vi "v6.0.vi"() -> ()   [LabVIEW 2018]
uses:
  <vilib>/DAQmx/read.llb/DAQmx Read (Analog 1D DBL NChan 1Samp).vi
  <extravilib>/ChannelInstances/Lossy Stream-c(a[.](c(dbl,dbl,dbl,dbl)),stamp,a[.](dbl),c(dbl,dbl,dbl,dbl,dbl,dbl,dbl))/Read With Abort.vi
  <extravilib>/ChannelInstances/High Speed Stream-c(a[.](c(dbl,dbl,dbl,dbl)),stamp,a[.](dbl),c(dbl,dbl,dbl,dbl,dbl,dbl,dbl))/_Read For Replicate.vi
  <extravilib>/ChannelInstances/Lossy Stream-c(a[.](c(dbl,dbl,dbl,dbl)),stamp,a[.](dbl),c(dbl,dbl,dbl,dbl,dbl,dbl,dbl))/Write With Abort.vi
  <extravilib>/ChannelInstances/Lossy Stream-c(a[.](c(dbl,dbl,dbl,dbl)),stamp,a[.](dbl),c(dbl,dbl,dbl,dbl,dbl,dbl,dbl))/EndpointRead.vi
  <extravilib>/ChannelInstances/Lossy Stream-c(a[.](c(dbl,dbl,dbl,dbl)),stamp,a[.](dbl),c(dbl,dbl,dbl,dbl,dbl,dbl,dbl))/Endpoint.vi
  <extravilib>/ChannelInstances/Lossy Stream-c(a[.](c(dbl,dbl,dbl,dbl)),stamp,a[.](dbl),c(dbl,dbl,dbl,dbl,dbl,dbl,dbl))/Instantiate.vi
  <extravilib>/ChannelInstances/Lossy Stream-c(a[.](c(dbl,dbl,dbl,dbl)),stamp,a[.](dbl),c(dbl,dbl,dbl,dbl,dbl,dbl,dbl))/)Channel.vi
  <resource>/ChannelSupport/_ChannelSupport/WaitIfNeeded.vi
  <extravilib>/ChannelInstances/High Speed Stream-c(a[.](c(dbl,dbl,dbl,dbl)),stamp,a[.](dbl),c(dbl,dbl,dbl,dbl,dbl,dbl,dbl))/Instantiate.vi
  <extravilib>/ChannelInstances/High Speed Stream-c(a[.](c(dbl,dbl,dbl,dbl)),stamp,a[.](dbl),c(dbl,dbl,dbl,dbl,dbl,dbl,dbl))/)Channel.vi
  <extravilib>/ChannelInstances/High Speed Stream-c(a[.](c(dbl,dbl,dbl,dbl)),stamp,a[.](dbl),c(dbl,dbl,dbl,dbl,dbl,dbl,dbl))/Abort Signal/Init Signal.vi
  <vilib>/Utility/file.llb/Write Delimited Spreadsheet (string).vi
  <vilib>/DAQmx/create/channels.llb/DAQmx Create Channel (AI-Temperature-Thermocouple).vi
  <vilib>/DAQmx/configure/timing.llb/DAQmx Timing (Sample Clock).vi
  <vilib>/DAQmx/miscellaneous.llb/DAQmx Fill In Error Info.vi
  <extravilib>/ChannelInstances/High Speed Stream-c(a[.](c(dbl,dbl,dbl,dbl)),stamp,a[.](dbl),c(dbl,dbl,dbl,dbl,dbl,dbl,dbl)).lvlib
  <resource>/objmgr/daqmx.rc
  <extravilib>/ChannelInstances/Lossy Stream-c(a[.](c(dbl,dbl,dbl,dbl)),stamp,a[.](dbl),c(dbl,dbl,dbl,dbl,dbl,dbl,dbl)).lvlib
panel:
  in  "Line Controls\n(Don't Delete)":enum32{"Flowrate", "Temperatures", "Pressures"}(tab)
  in  "Line Flowrate Control":T1 {"Line 5" scale=0.0..10.0; "Line 4" scale=0.0..10.0; "Line 3" scale=0.0..10.0; "Line 2" scale=0.0..10.0; "Line 1" scale=0.0..10.0}
  in  "Temperatures Control":T1 {"Line 5" scale=0.0..10.0; "Line 4" scale=0.0..10.0; "Line 3" scale=0.0..10.0; "Line 2" scale=0.0..10.0; "Line 1" scale=0.0..10.0}
  in  "Pressure Controls":T1 {"Line 5" scale=0.0..10.0; "Line 4" scale=0.0..10.0; "Line 3" scale=0.0..10.0; "Line 2" scale=0.0..10.0; "Line 1" scale=0.0..10.0}
  out "Thermal Power [kJ/s]":dbl
  out "Equivalence Ratio":dbl
  out "Total Air Flow Required for \nStoichiometric Combustion":dbl
  out "Mixture AFR":dbl
  out "Total Fuel Flow [g/s]":dbl
  out "Total Air Flow [g/s]":dbl
  in  "Rig Temperature Tab Box\n(Don't Delete)":enum32{"Rig Temps Live", "Alarm Thresholds"}(tab)
  out "Rig Temperatures":T2
  in  "Rig Alarm Thresholds":T2
  out "DAQ Current Time":timestamp format="%<%X>T"
  in  "UI Refresh Rate (Hz)":u32=1 min=1 max=500 step=1
  out "Line Pressures":T3(graph)
  out "Line Temperatures":T3(graph)
  in  "Species List":string[][](table)=[["Custom", "9999999999", ""], ["Methanol", "6.47", "19.93"], ["Butanol", "11.2", "33.075"], ["Propane", "15.67", "46.35"], ["Methane", "13.19", "50.00"], ["Hydrogen", "34.3", "119.96"], ["Ammonia", "6.0466", "22.5"], ["Pentane", "15.32", "45.36"], ["Butane", "14.98", "45.75"], ["Hexane", "15.24", "44.75"], ["Ethanol", "9", "26.70"], ["Empty (Not Used)", "0", "0"]]
  in  "Lines Tab Control\n(Don't delete)":enum32{"Live Data", "AFR Info", "Setup Lines"}(tab)
  out "Flowrate Data":T4(array[cluster])
  out "AFR Display":T5(array[cluster])
  in  "Line Setup":T6(array[cluster])
  out "Actual Sample Rate":dbl
  out "Export Timestamp":timestamp format="%<%H:%M:%S>T"
  out "UI Timestamp":timestamp format="%<%X\n%x>T"
  in  "file path (dialog if empty)":path
  out "Export Loop Status":T7(ring)
  in  "Start Recording?":bool
  in  "Stop Recording?":bool
  out "Aquisition\nLoop Status":T8(ring)
  in  "OK Button":bool
  in  "DAQ Properties":cluster{"Sample Rate [Hz]":dbl}={"Sample Rate [Hz]"=1.0} {"Sample Rate [Hz]" min=1.0 max=500.0 step=1.0}
  # "Rig Temperatures [ °C]"
  # "Rig Alarm Thresholds [ °C]"
  # "Live \n Live Line Data"
  # "Air-to-Fuel Ratios for each Line"
  # "Line Setup"
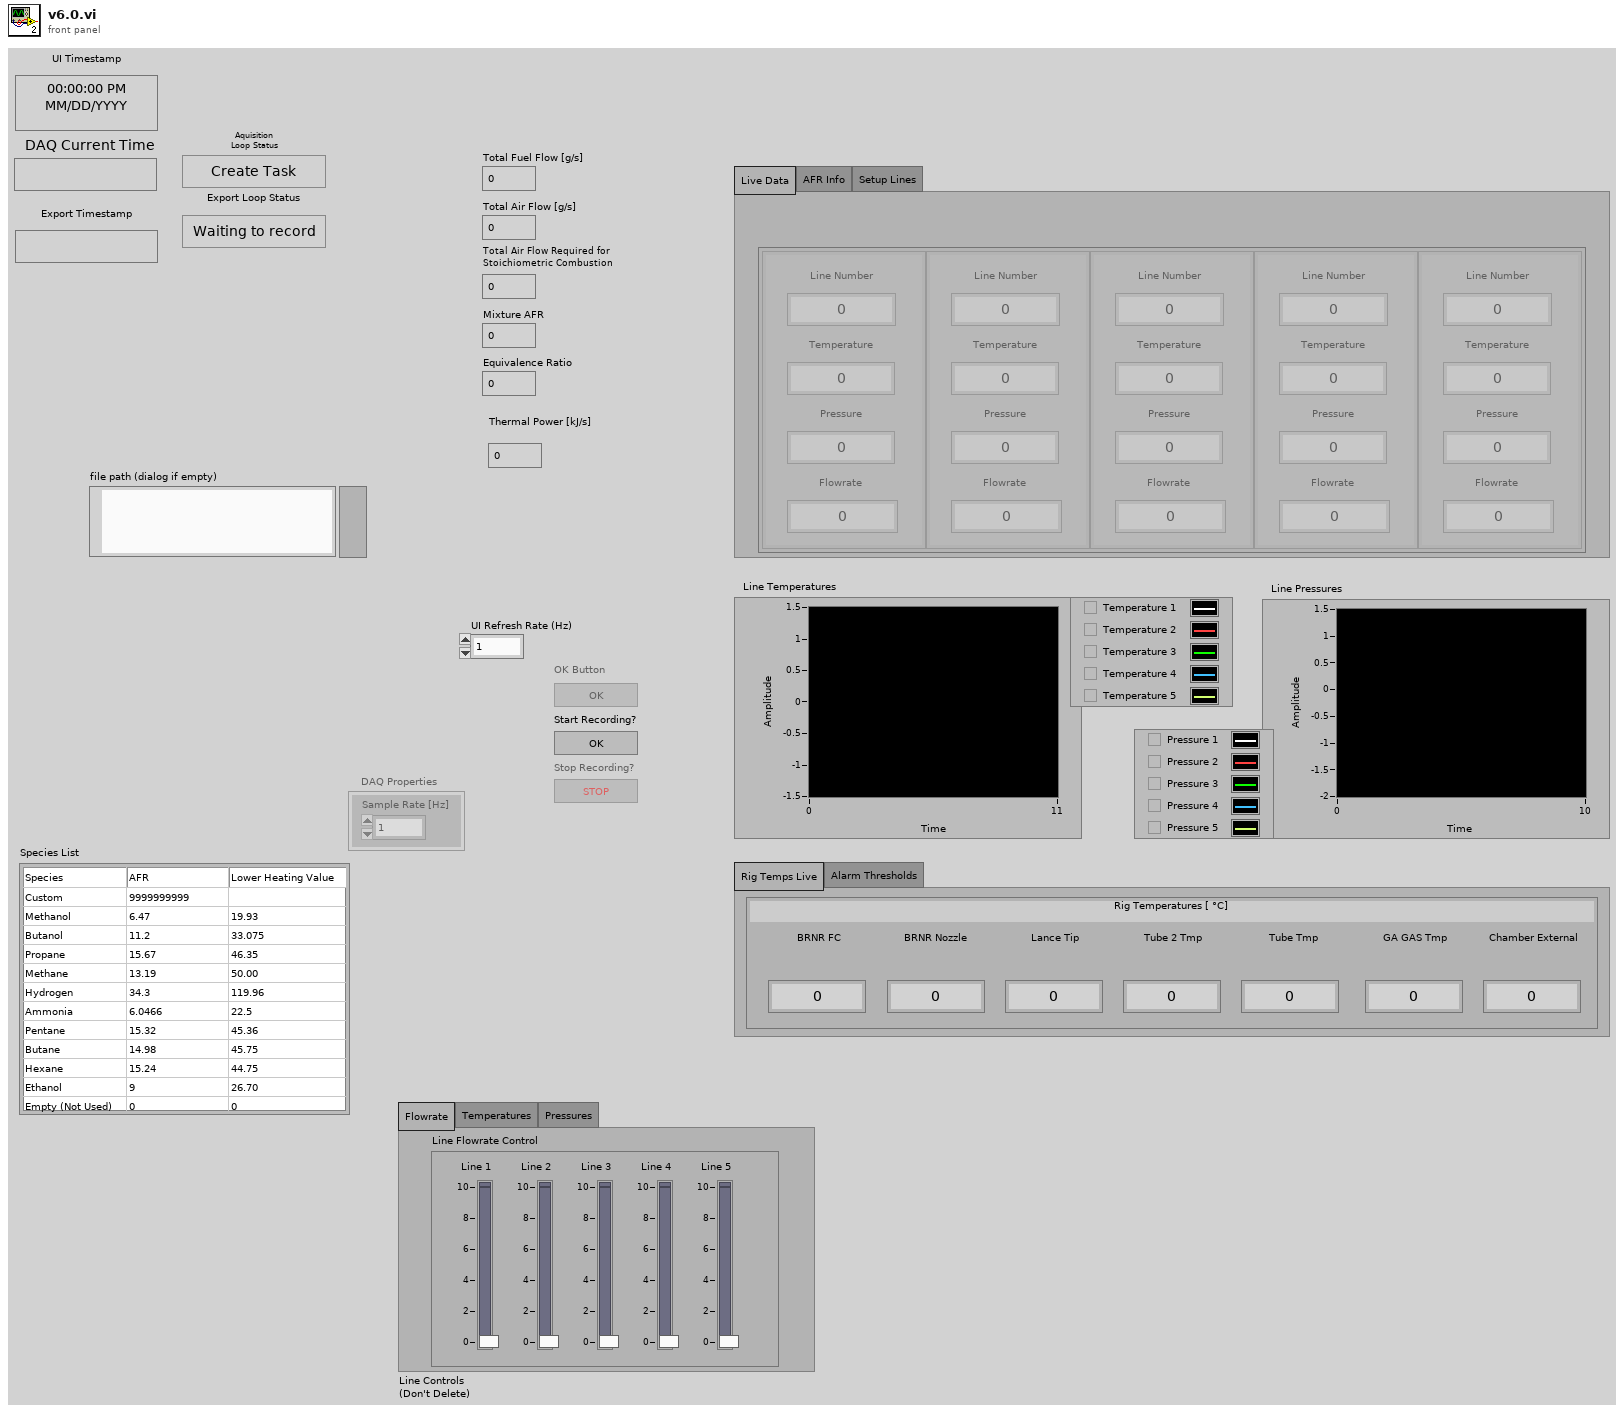
[diagram p1: front panel]
types:
  T1 = cluster{"Line 1":dbl, "Line 2":dbl, "Line 3":dbl, "Line 4":dbl, "Line 5":dbl}
  T2 = cluster{"BRNR FC":dbl, "BRNR Nozzle":dbl, "Lance Tip":dbl, "Tube 2 Tmp":dbl, "Tube Tmp":dbl, "GA GAS Tmp":dbl, "Chamber External":dbl}
  T3 = cluster{"[0]":dbl, "[1]":dbl, "[2]":dbl, "[3]":dbl, "[4]":dbl}
  T4 = cluster{"Line Number":dbl, "Temperature":dbl, "Pressure":dbl, "Flowrate":dbl}[]
  T5 = cluster{"Line Number":i32, "AFR":dbl, "Species":enum16{"Empty (Not used)", "Custom", "Air", "Methanol", "Ethanol", "Butanol", "Propane", "Methane", "Hydrogen", "Pentane", "Butane", "Hexane"}}[]
  T6 = cluster{"Custom AFR":dbl, "Species":enum16{"Empty (Not used)", "Custom", "Air", "Methanol", "Ethanol", "Butanol", "Propane", "Methane", "Hydrogen", "Pentane", "Butane", "Hexane"}, "Custom Lower Heating Value [kJ/kg]":dbl}[]
  T7 = enum16{"Waiting to record", "Creating Spreadsheet", "Recording", "Finished Recording"}
  T8 = enum16{"Create Task", "Change Settings", "Check Settings", "Read Data", "End Task"}
  T9 = enum8{"Enabled", "Disabled", "Disabled and Grayed Out"}
  T10 = cluster{"Flowrate Data":cluster{"Line Number":dbl, "Temperature":dbl, "Pressure":dbl, "Flowrate":dbl}[], "Current Time":timestamp, "DAQmx Data":dbl[], "Rig Temperatures":cluster{"BRNR FC":dbl, "BRNR Nozzle":dbl, "Lance Tip":dbl, "Tube 2 Tmp":dbl, "Tube Tmp":dbl, "GA GAS Tmp":dbl, "Chamber External Temp":dbl}}
  T11 = cluster{"BRNR FC":dbl, "BRNR Nozzle":dbl, "Lance Tip":dbl, "Tube 2 Tmp":dbl, "Tube Tmp":dbl, "GA GAS Tmp":dbl, "Chamber External Temp":dbl}
  T12 = typedef "High Speed Stream-c(a[.](c(dbl,dbl,dbl,dbl)),stamp,a[.](dbl),c(dbl,dbl,dbl,dbl,dbl,dbl,dbl)).lvlib/)Channel.ctl" = refnum<queue>
  T13 = typedef "Lossy Stream-c(a[.](c(dbl,dbl,dbl,dbl)),stamp,a[.](dbl),c(dbl,dbl,dbl,dbl,dbl,dbl,dbl)).lvlib/)Channel.ctl" = refnum<queue>
  T14 = cluster{"Line":i32, "AFR":dbl, "Species":enum16{"Empty (Not used)", "Custom", "Air", "Methanol", "Ethanol", "Butanol", "Propane", "Methane", "Hydrogen", "Pentane", "Butane", "Hexane"}}
  T15 = enum16{"Empty (Not used)", "Custom", "Air", "Methanol", "Ethanol", "Butanol", "Propane", "Methane", "Hydrogen", "Pentane", "Butane", "Hexane"}
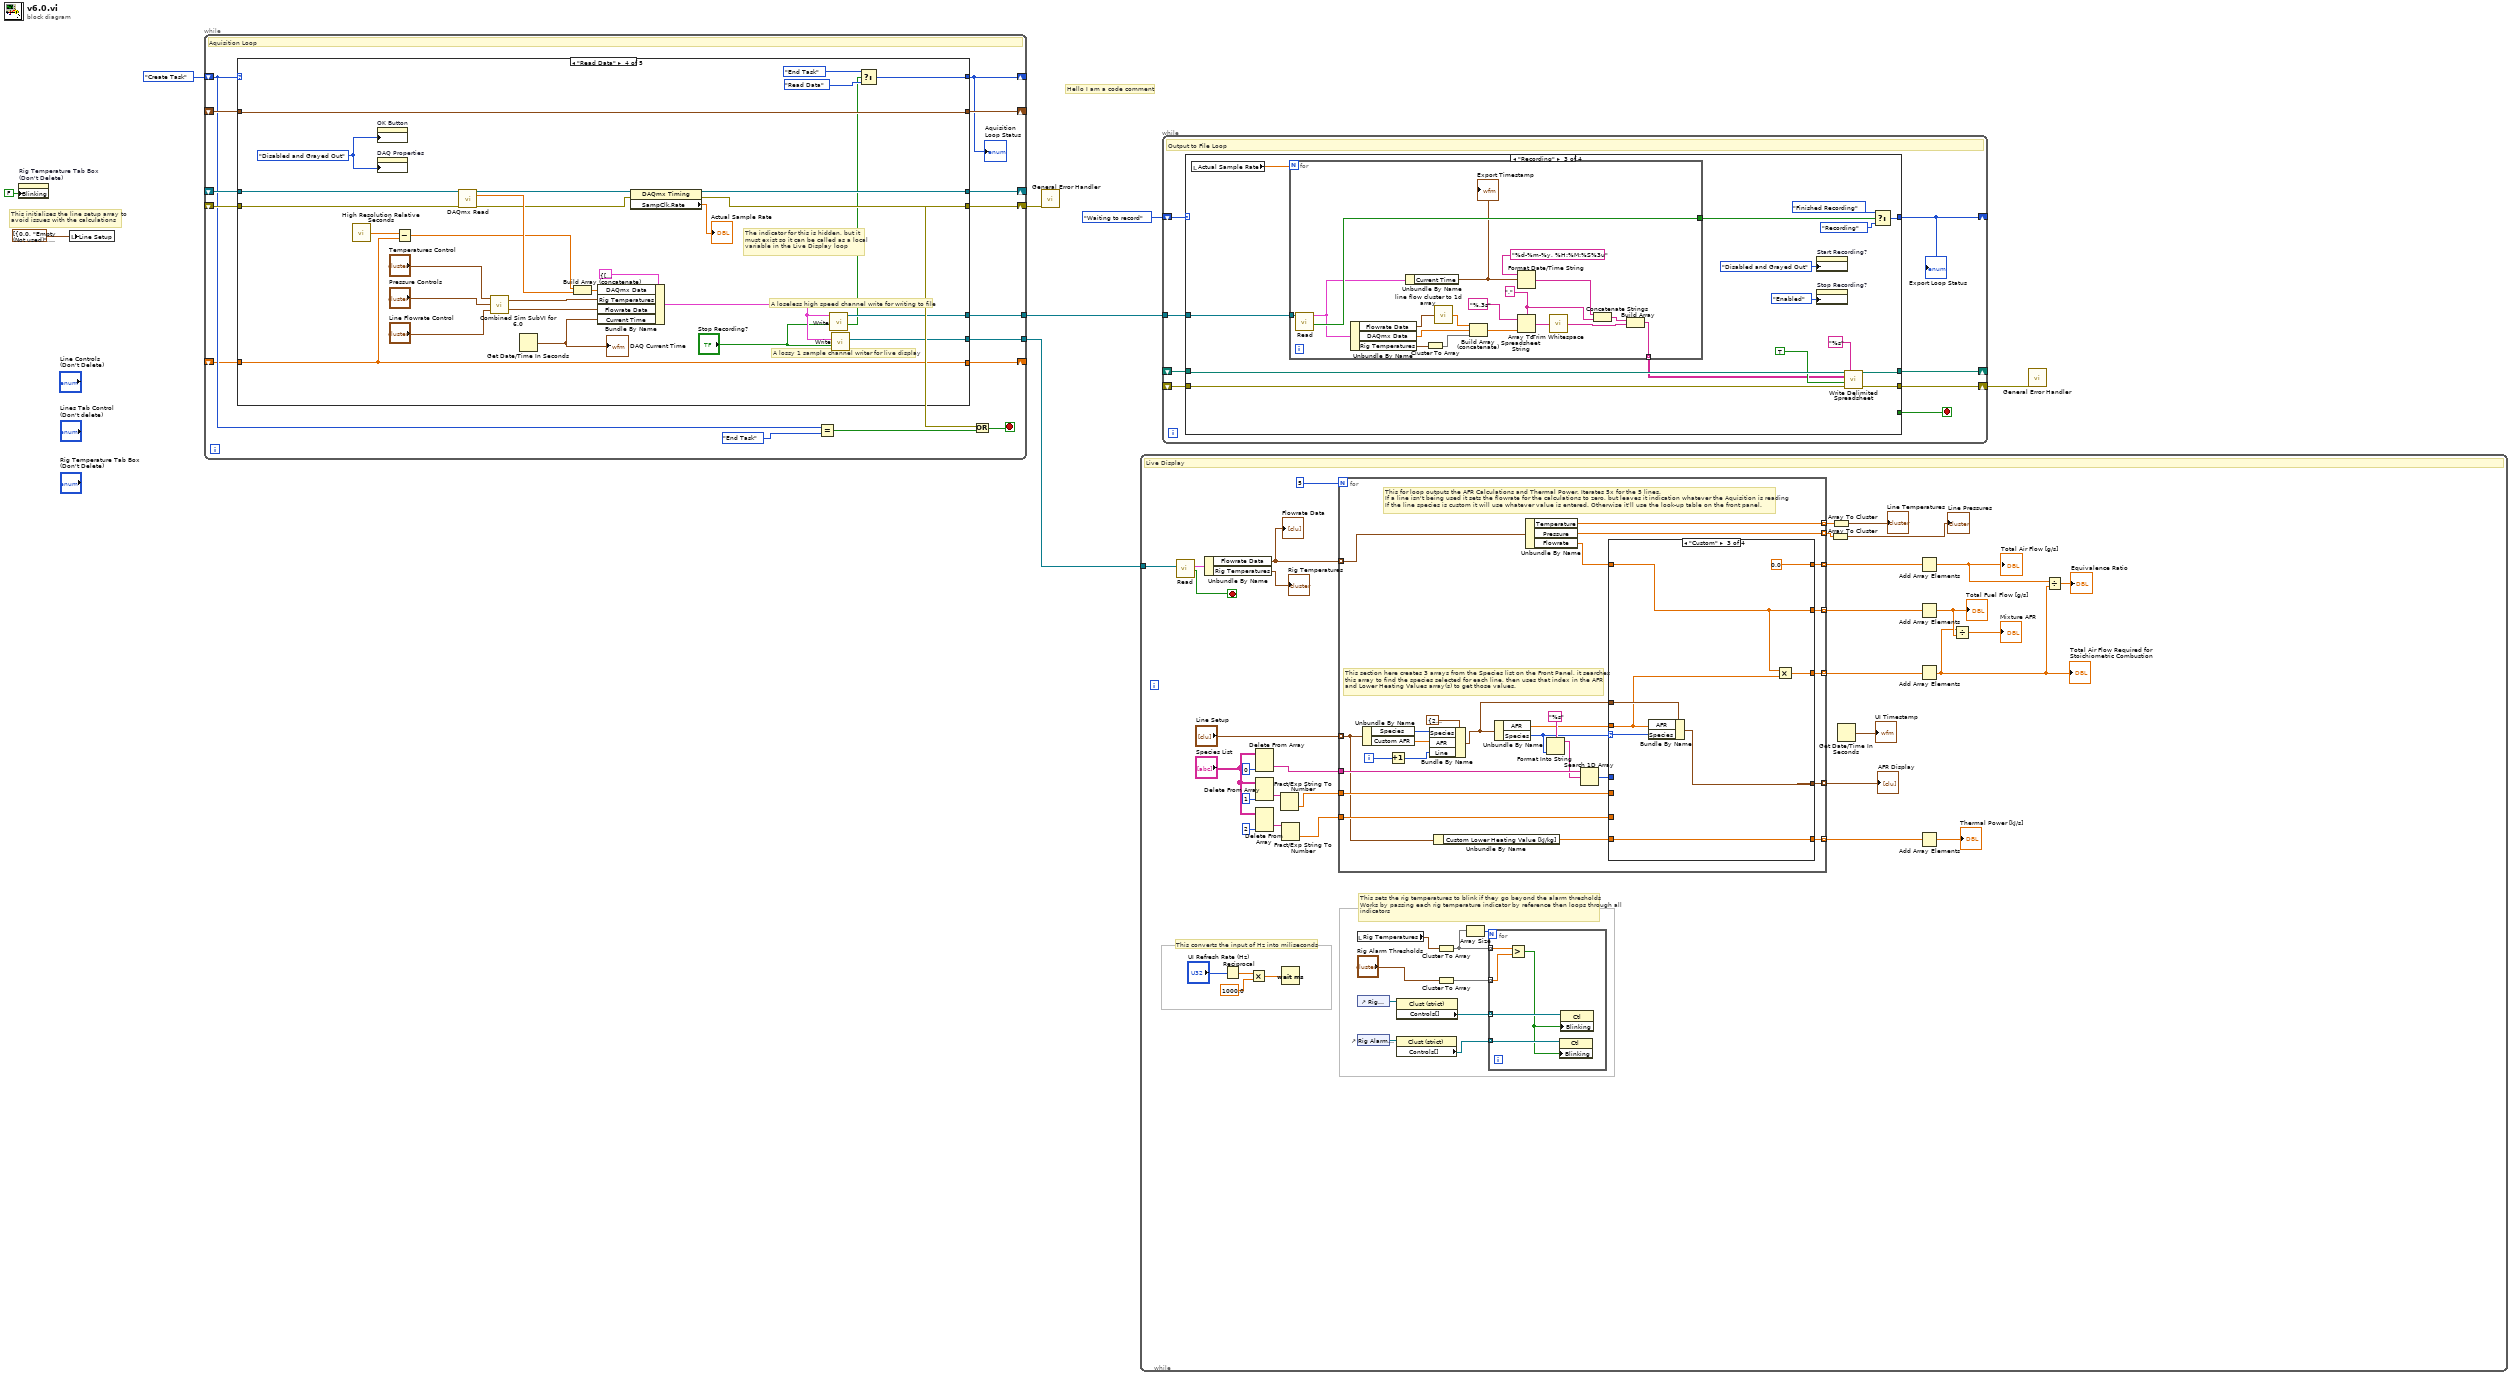
[diagram p0: block diagram]
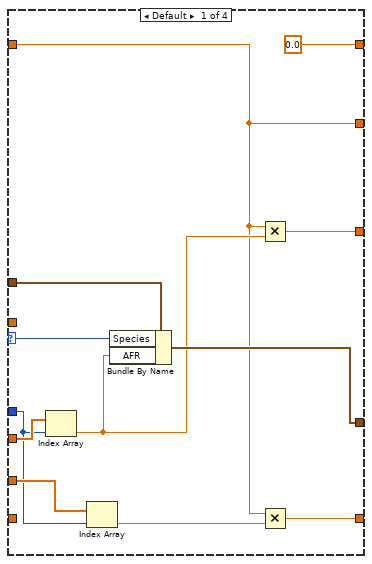
[diagram p2: hidden frame]
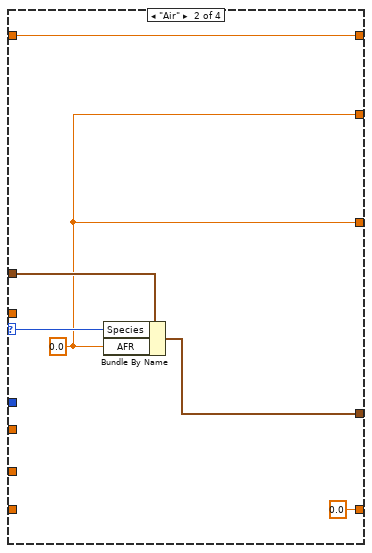
[diagram p3: hidden frame]
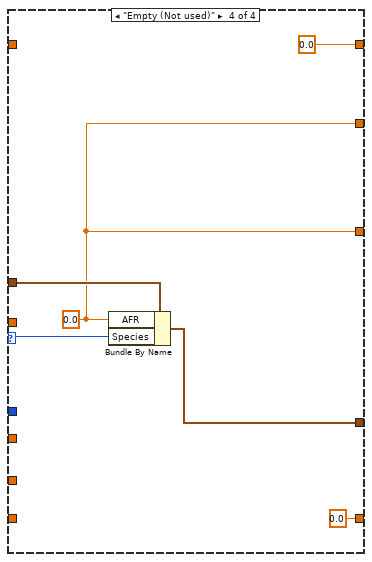
[diagram p4: hidden frame]
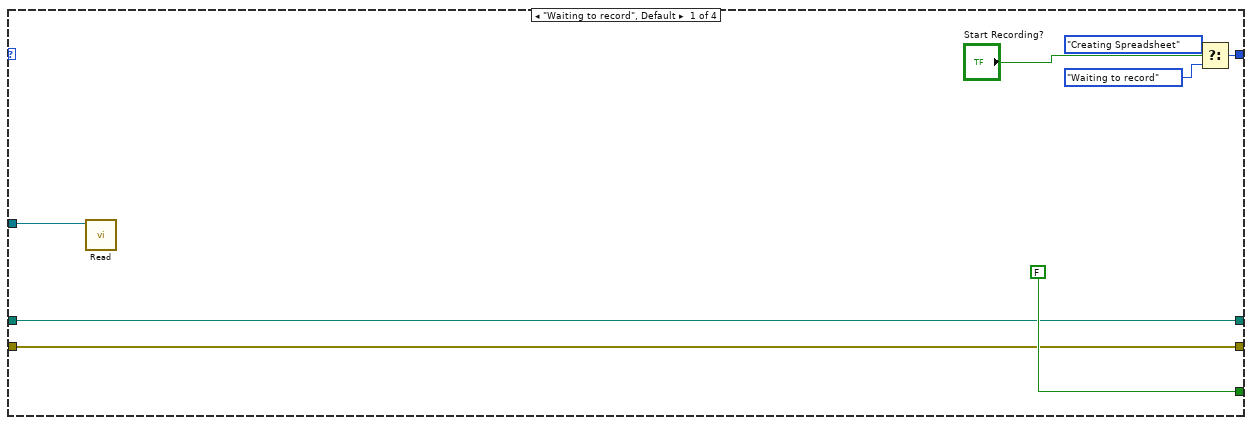
[diagram p5: hidden frame]
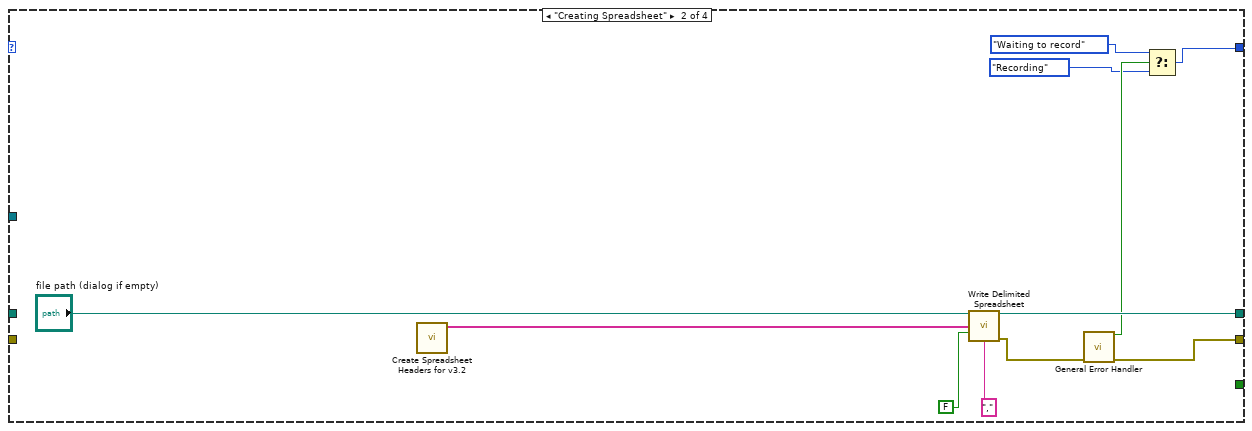
[diagram p6: hidden frame]
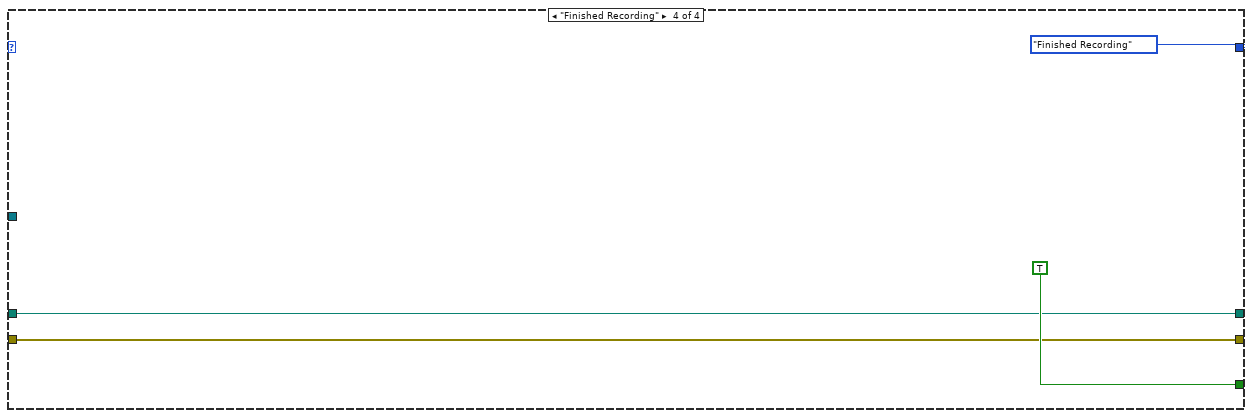
[diagram p7: hidden frame]
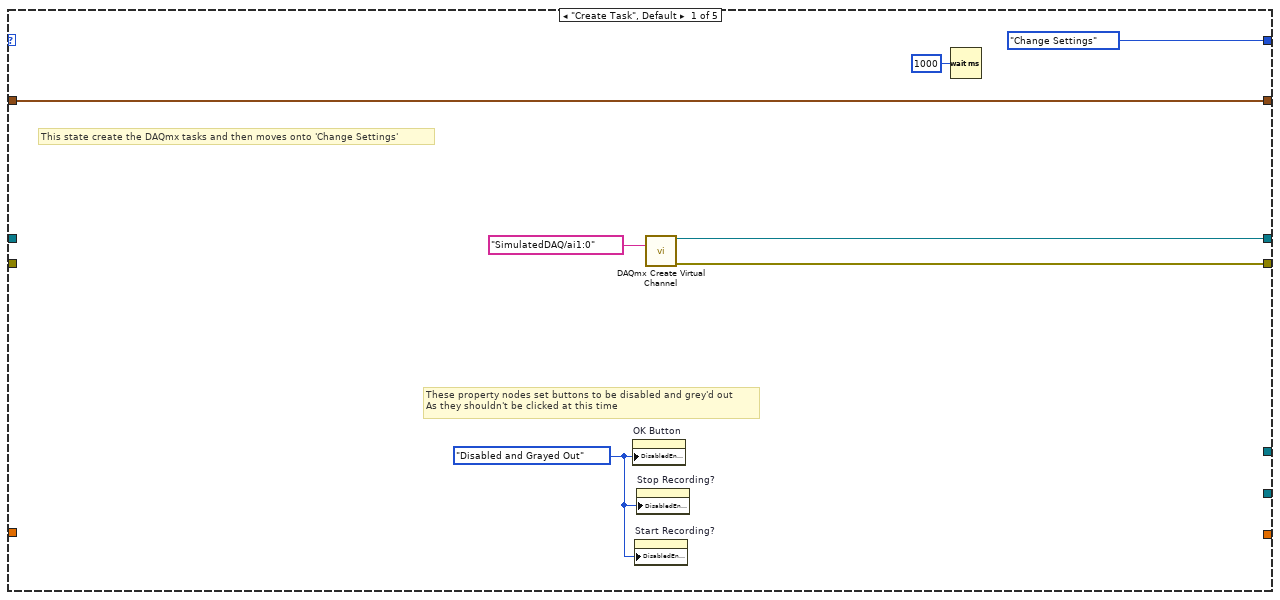
[diagram p8: hidden frame]
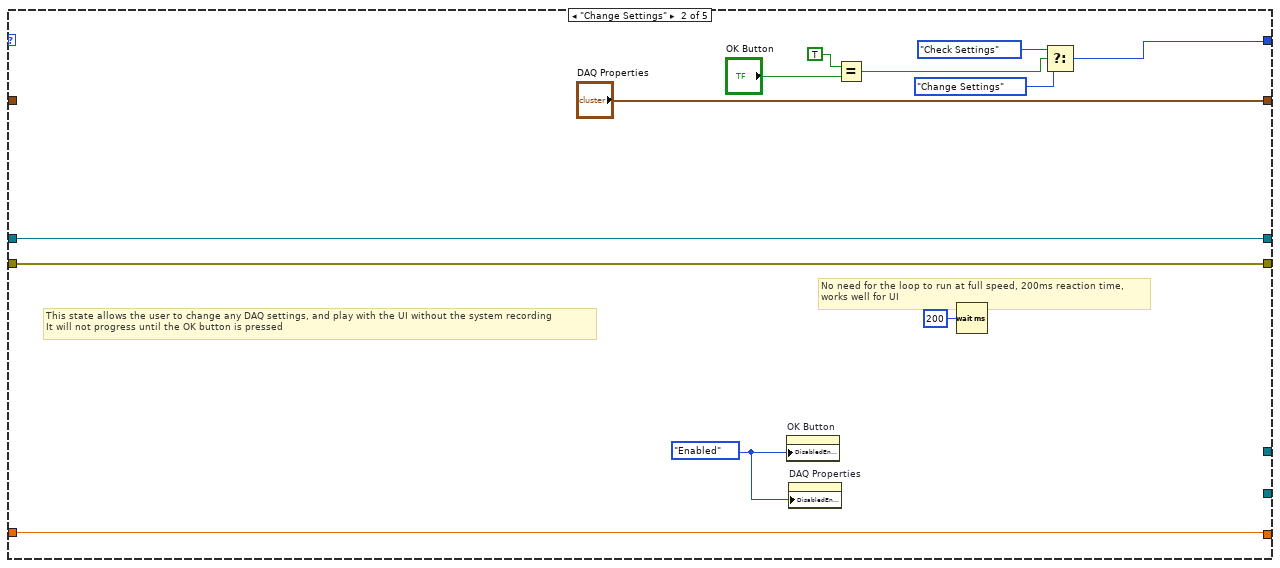
[diagram p9: hidden frame]
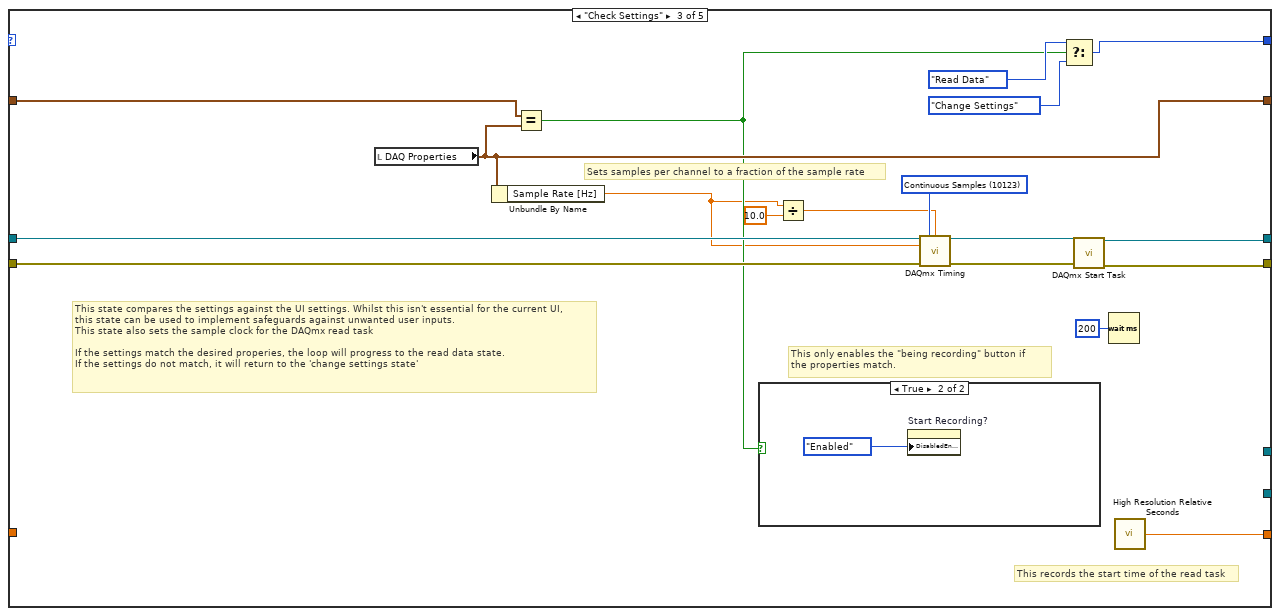
[diagram p10: hidden frame]
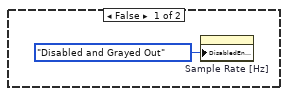
[diagram p11: hidden frame]
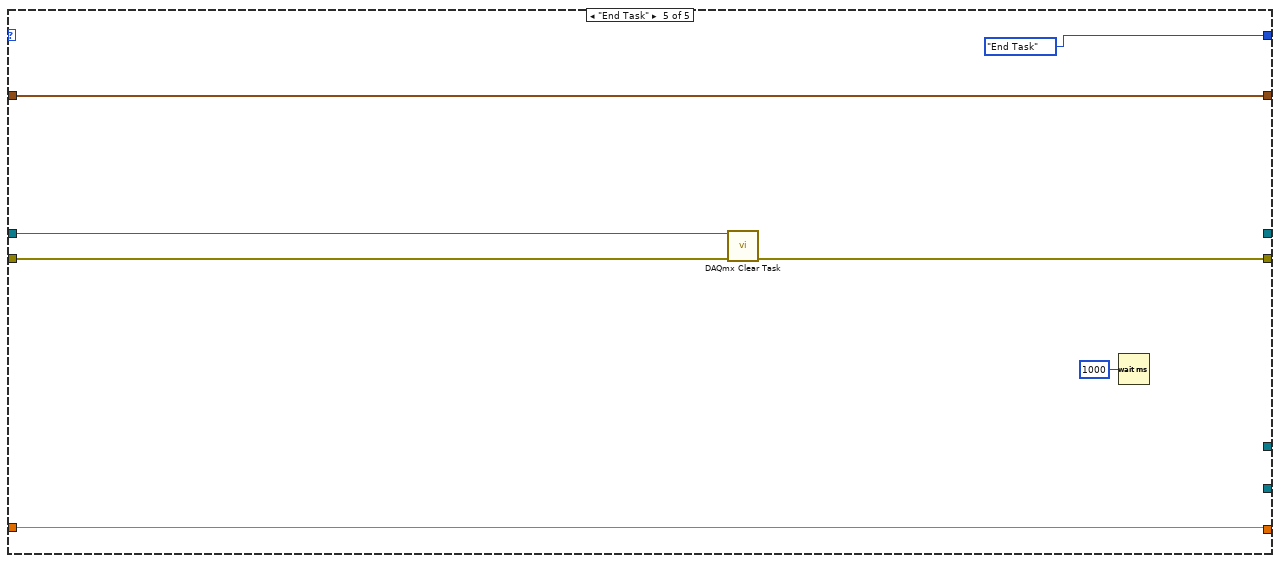
[diagram p12: hidden frame]
diagram:
  # "Hello I am a code comment"
  # "This initialises the line setup array to\navoid issues with the calculations"
  n1 = property on="Rig Temperature Tab Box\n(Don't Delete)" class="TabCtl (strict)"("Blinking"=FALSE) -> ()  [unwired: 2 in, 2 out]
  n2 = local write "Line Setup"(T6 [{"Custom AFR"=0.0, "Species"=enum."Empty (Not used)", "Custom Lower Heating Value [kJ/kg]"=0.0}, {"Custom AFR"=0.0, "Species"=enum."Empty (Not used)", "Custom Lower Heating Value [kJ/kg]"=0.0}, {"Custom AFR"=0.0, "Species"=enum."Empty (Not used)", "Custom Lower Heating Value [kJ/kg]"=0.0}, {"Custom AFR"=0.0, "Species"=enum."Empty (Not used)", "Custom Lower Heating Value [kJ/kg]"=0.0}, {"Custom AFR"=0.0, "Species"=enum."Empty (Not used)", "Custom Lower Heating Value [kJ/kg]"=0.0}] ("Line Setup")) -> ()
  n3 = while {
    shift-right: [w18] -> _
    shift-left: T8."Create Task" -> [w14]
    shift-right: [w23] -> _
    shift-left: _ -> [w21]
    shift-right: [w17] -> w4
    shift-left: _ -> [w20]
    shift-right: [w22] -> _
    shift-left: _ -> [w19]
    tunnel: [w13] -> w6
    tunnel: [w11] -> w3
    shift-right: [w9] -> _
    shift-left: _ -> [w10]
    stop <- w12 stop-if-true
    # "Aquisition Loop"
    n4 = case shown="\"Read Data\"" w14 {
      tunnel: [w30 w42 w50 w78 _] -> w23
      tunnel: [w29 w41 w49 w79 w98] -> w17
      tunnel: [T8."Change Settings" w35 w56 w87 T8."End Task"] -> w18
      tunnel: [w26 "DAQ Properties" w53 w89 w97] -> w22
      tunnel: w21 -> [_ w42 w55 w91 w95]
      tunnel: w20 -> [_ w41 w54 w90 w94]
      tunnel: w19 -> [w26 _ w60 w89 w97]
      tunnel: [_ _ _ w83 _] -> w13
      tunnel: [_ w31 w43 w74 w92] -> w9
      tunnel: w10 -> [_ w31 _ w74 w92]
      tunnel: [_ _ _ w71 _] -> w11
      frame "Create Task", Default {
        w24 = T9."Disabled and Grayed Out" ("Disabled")
        # "These property nodes set buttons to be disabled and grey'd out\nAs they shouldn't be clicked at this time"
        # "This state create the DAQmx tasks and then moves onto 'Change Settings'"
        n5 = property on="OK Button" class="Bool"("DisabledEnum"=w24) -> ()  [unwired: 2 in, 2 out]
        n6 = property on="Start Recording?" class="Bool"("DisabledEnum"=w24) -> ()  [unwired: 2 in, 2 out]
        n7 = property on="Stop Recording?" class="Bool"("DisabledEnum"=w24) -> ()  [unwired: 2 in, 2 out]
        n8 = call-poly <vilib>:"DAQmx Create Virtual Channel.vi"("physical channels"=tag "SimulatedDAQ/ai1:0") -> ("task out"=w30:refnum<k21>, "error out"=w29:errorcluster)  [unwired: 13 in]
        n9 = Wait (ms)(milliseconds to wait=u32 1000) -> ()  [unwired: 1 out]
      }
      frame "Change Settings" {
        w32 = T9."Enabled" ("Disabled")
        # "No need for the loop to run at full speed, 200ms reaction time,\nworks well for UI"
        # "This state allows the user to change any DAQ settings, and play with the UI without the system recording\nIt will not progress until the OK button is pressed"
        n10 = property on="OK Button" class="Bool"("DisabledEnum"=w32) -> ()  [unwired: 2 in, 2 out]
        n11 = property on="DAQ Properties" class="Clust (strict)"("DisabledEnum"=w32) -> ()  [unwired: 2 in, 2 out]
        n12 = Equal?(x=TRUE, y="OK Button") -> (x = y?=w37:bool)
        n13 = Wait (ms)(milliseconds to wait=u32 200) -> ()  [unwired: 1 out]
        n14 = Select(t=T8."Check Settings", s=w37, f=T8."Change Settings") -> (s? t:f=w35:T8)
      }
      frame "Check Settings" {
        w48 = 10123 items=["Finite Samples"=10178, "Continuous Samples"=10123, "Hardware Timed Single Point"=12522] ("sample mode")
        # "This records the start time of the read task"
        # "This only enables the \"being recording\" button if \nthe properties match."
        # "Sets samples per channel to a fraction of the sample rate"
        # "This state compares the settings against the UI settings. Whilst this isn't essential for the current UI, \nthis state can be used to implement safeguards against unwanted user inputs.\nThis state also sets the sample clock for the DAQmx read task\n\nIf the settings match the desired properies, the loop will progress to the read data state.\nIf the settings do not match, it will return to the 'change settings state'"
        n15 = local read "DAQ Properties"() -> (w53:cluster{"Sample Rate [Hz]":dbl})
        n16 = Unbundle By Name(w53) -> ("Sample Rate [Hz]"=w45:dbl)
        n17 = Equal?(x=w60, y=w53) -> (x = y?=w47:bool)
        n18 = case shown="True" w47 {
          frame False {
            n19 = property on="Sample Rate [Hz]" class="DigNum (strict)"("DisabledEnum"=T9."Disabled and Grayed Out" ("Disabled")) -> ()  [unwired: 2 in, 2 out]
          }
          frame True {
            n20 = property on="Start Recording?" class="Bool"("DisabledEnum"=T9."Enabled" ("Disabled")) -> ()  [unwired: 2 in, 2 out]
          }
        }
        n21 = Divide(x=w45, y=10.0) -> (x/y=w44:dbl)
        n22 = call-poly <vilib>:"DAQmx Timing.vi"("task/channels in"=w55, "sample mode"=w48, "samples per channel"=w44, "rate"=w45, "error in"=w54) -> ("task out"=w52:refnum<k21>, "error out"=w51:errorcluster)  [unwired: 9 in]
        n23 = Select(t=T8."Read Data", s=w47, f=T8."Change Settings") -> (s? t:f=w56:T8)
        n24 = call <vilib>:"DAQmx Start Task.vi"("task/channels in"=w52, "error in"=w51) -> ("task out"=w50:refnum<k21>, "error out"=w49:errorcluster)  [unwired: 12 in]
        n25 = Wait (ms)(milliseconds to wait=u32 200) -> ()  [unwired: 1 out]
        n26 = call <vilib>:"High Resolution Relative Seconds.vi"() -> ("relative seconds"=w43:dbl)
      }
      frame "Read Data" {
        w82 = T9."Disabled and Grayed Out" ("Disabled")
        # "A lossy 1 sample channel writer for live display"
        # "A loseless high speed channel write for writing to file"
        # "The indicator for this is hidden, but it\nmust exist so it can be called as a local \nvariable in the Live Display loop"
        n27 = call <vilib>:"High Resolution Relative Seconds.vi"() -> ("relative seconds"=w76:dbl)
        n28 = property on="OK Button" class="Bool"("DisabledEnum"=w82) -> ()  [unwired: 2 in, 2 out]
        n29 = property on="DAQ Properties" class="Clust (strict)"("DisabledEnum"=w82) -> ()  [unwired: 2 in, 2 out]
        n30 = Subtract(x=w76, y=w74) -> (x-y=w75:dbl)
        n31 = call-poly <vilib>:"DAQmx Read.vi"("task/channels in"=w91, "error in"=w90) -> ("task out"=w80:refnum<k21>, "data"=w85:dbl[], "error out"=w77:errorcluster)  [unwired: 11 in]
        n32 = call "Combined Sim SubVI for 6.0.vi"("Pressure Controls"="Line Flowrate Control", "Line Flowrate Control"="Pressure Controls", "Temperatures Control"="Temperatures Control") -> ("Array"=w63:T4, "Cluster"=w64:T11)
        n33 = Get Date/Time In Seconds() -> (seconds since 1Jan1904=w68:timestamp)
        "DAQ Current Time" <- w68
        n34 = Build Array (concatenate)(w75, w85) -> (w69:dbl[])
        n35 = Bundle By Name(cluster=T10 {"Flowrate Data"=[{"Line Number"=1.0, "Temperature"=17.480721541683437, "Pressure"=24.0, "Flowrate"=0.0}, {"Line Number"=2.0, "Temperature"=21.850901927104296, "Pressure"=30.0, "Flowrate"=0.0}, {"Line Number"=3.0, "Temperature"=26.221082312525155, "Pressure"=36.0, "Flowrate"=0.0}, {"Line Number"=4.0, "Temperature"=30.591262697946018, "Pressure"=42.00000000000001, "Flowrate"=0.0}, {"Line Number"=5.0, "Temperature"=34.96144308336687, "Pressure"=48.0, "Flowrate"=0.0}], "Current Time"=timestamp(0 s since 1904-01-01), "DAQmx Data"=[], "Rig Temperatures"={"BRNR FC"=0.0, "BRNR Nozzle"=0.0, "Lance Tip"=0.0, "Tube 2 Tmp"=0.0, "Tube Tmp"=0.0, "GA GAS Tmp"=0.0, "Chamber External Temp"=0.0}}, "DAQmx Data"=w69, "Rig Temperatures"=w64, "Flowrate Data"=w63, "Current Time"=w68) -> (w81:T10)
        n36 = property class="DAQmx Timing"(reference=w80, error in=w77) -> (reference out=w78:refnum<k21>, error out=w79:errorcluster, "SampClk.Rate"=→"Actual Sample Rate":dbl)
        n37 = call <extravilib>:"Write.vi"("last element? (F)"="Stop Recording?", "element"=w81) -> ("done?"=w70:bool, "channel"=w83:T12)  [unwired: 7 in, 1 out]
        n38 = call <extravilib>:"Write.vi"("last element? (F)"="Stop Recording?", "element"=w81) -> ("channel"=w71:T13)  [unwired: 7 in, 2 out]
        n39 = Select(t=T8."End Task", s=w70, f=T8."Read Data") -> (s? t:f=w87:T8)
      }
      frame "End Task" {
        n40 = call <vilib>:"DAQmx Clear Task.vi"("task in"=w95, "error in"=w94) -> ("error out"=w98:errorcluster)  [unwired: 13 in]
        n41 = Wait (ms)(milliseconds to wait=u32 1000) -> ()  [unwired: 1 out]
      }
    }
    "Aquisition\nLoop Status" <- w18
    n42 = Equal?(x=w14, y=T8."End Task") -> (x = y?=w15:bool)
    n43 = Or(x=w17, y=w15) -> (x .or. y?=w12:bool)
  }
  n44 = call <vilib>:"General Error Handler.vi"("error in (no error)"=w4) -> ()  [unwired: 10 in, 5 out]
  n45 = while {
    tunnel: w3 -> [w142]
    stop <- w139 stop-if-true
    # "This converts the input of Hz into miliseconds"
    # "This sets the rig temperatures to blink if they go beyond the alarm thresholds\nWorks by passing each rig temperature indicator by reference then loops through all indicators"
    # "Live Display"
    n46 = call <extravilib>:"Read.vi"("channel"=w142) -> ("last element?"=w139:bool, "element"=w141:T10)  [unwired: 5 in, 4 out]
    n47 = Unbundle By Name(w141) -> ("Flowrate Data"=w119:T4, "Rig Temperatures"=→"Rig Temperatures":T11)
    "Flowrate Data" <- w119
    n48 = Reciprocal(x="UI Refresh Rate (Hz)") -> (1/x=w100:dbl)
    n49 = Multiply(x=w100, y=1000.0) -> (x*y=w137:dbl)
    n50 = Delete From Array(array="Species List", index (col)=0) -> (deleted portion=w132:string[])  [unwired: 2 in, 1 out]
    n51 = Delete From Array(array="Species List", index (col)=1 ("disabled index (col)")) -> (deleted portion=w133:string[])  [unwired: 2 in, 1 out]
    n52 = Delete From Array(array="Species List", index (col)=2 ("disabled index (col)")) -> (deleted portion=w104:string[])  [unwired: 2 in, 1 out]
    n53 = Fract/Exp String To Number(string=w133) -> (number=w134:dbl[])  [unwired: 3 in, 1 out]
    n54 = Fract/Exp String To Number(string=w104) -> (number=w103:dbl[])  [unwired: 3 in, 1 out]
    n55 = Wait (ms)(milliseconds to wait=w137) -> ()  [unwired: 1 out]
    n56 = for {
      N: 5 -> [_]
      tunnel: w132 -> [w172]
      tunnel: w134 -> [w169]
      tunnel: "Line Setup" -> [w150] mode=indexing
      tunnel: [w160] -> w136 mode=indexing
      tunnel: w119 -> [w154] mode=indexing
      tunnel: [w159] -> w127 mode=indexing
      tunnel: [w158] -> w124 mode=indexing
      tunnel: [w156] -> w122 mode=indexing
      tunnel: [w155] -> w121 mode=indexing
      tunnel: [w153] -> w120 mode=indexing
      tunnel: w103 -> [w152]
      tunnel: [w151] -> w101 mode=indexing
      i -> [w162]
      # "This section here creates 3 arrays from the Species list on the Front Panel, it searches \nthis array to find the species selected for each line, then uses that index in the AFR \nand Lower Heating Values array(s) to get those values."
      # "This for loop outputs the AFR Calculations and Thermal Power. Iterates 5x for the 5 lines.\nIf a line isn't being used it sets the flowrate for the calculations to zero, but leaves it indication whatever the Aquisition is reading\nIf the line species is custom it will use whatever value is entered. Otherwise it'll use the look-up table on the front panel."
      n57 = Unbundle By Name(w150) -> ("Species"=w166:T15, "Custom AFR"=w165:dbl)
      n58 = Increment(x=w162) -> (x+1=w163:i32)
      n59 = Bundle By Name(cluster=T14 {"Line"=2, "AFR"=1.0, "Species"=enum."Butane"} ("AFR Inputs"), "Species"=w166, "AFR"=w165, "Line"=w163) -> (w161:T14)
      n60 = Unbundle By Name(w150) -> ("Custom Lower Heating Value [kJ/kg]"=w149:dbl)
      n61 = Unbundle By Name(w161) -> ("AFR"=w170:dbl, "Species"=w167:T15)
      n62 = Unbundle By Name(w154) -> ("Temperature"=w159:dbl, "Pressure"=w158:dbl, "Flowrate"=w157:dbl)
      n63 = Format Into String(format string="%s", w167) -> (resulting string=w171:string)  [unwired: 2 in, 1 out]
      n64 = Search 1D Array(1D array=w172, element=w171) -> (index of element=w168:i32)  [unwired: 1 in]
      n65 = case shown="\"Custom\"" w167 {
        selector: w167 -> [w184 w191 w197 w203]
        tunnel: w170 -> [_ _ w195 _]
        tunnel: w169 -> [w185 _ _ _]
        tunnel: w168 -> [w177 _ _ _]
        tunnel: [w182 w190 w199 w205] -> w160
        tunnel: w161 -> [w183 w189 w198 w204]
        tunnel: w157 -> [w176 w188 w193 _]
        tunnel: [w180 w187 w194 w202] -> w156
        tunnel: [w176 w187 w193 w202] -> w155
        tunnel: [0.0 ("Flowrate") w188 0.0 ("Flowrate") 0.0 ("Flowrate")] -> w153
        tunnel: w152 -> [w178 _ _ _]
        tunnel: [w174 0.0 w192 0.0] -> w151
        tunnel: w149 -> [_ _ w192 _]
        frame Default {
          n66 = Index Array(array=w185, index=w177) -> (element=w181:dbl)
          n67 = Index Array(array=w178, index=w177) -> (element=w175:dbl)
          n68 = Bundle By Name(cluster=w183, "Species"=w184, "AFR"=w181) -> (w182:T14)
          n69 = Multiply(x=w176, y=w181) -> (x*y=w180:dbl)
          n70 = Multiply(x=w176, y=w175) -> (x*y=w174:dbl)
        }
        frame "Air" {
          w187 = 0.0 ("AFR")
          n71 = Bundle By Name(cluster=w189, "Species"=w191, "AFR"=w187) -> (w190:T14)
        }
        frame "Custom" {
          n72 = Bundle By Name(cluster=w198, "AFR"=w195, "Species"=w197) -> (w199:T14)
          n73 = Multiply(x=w193, y=w195) -> (x*y=w194:dbl)
        }
        frame "Empty (Not used)" {
          w202 = 0.0 ("AFR")
          n74 = Bundle By Name(cluster=w204, "AFR"=w202, "Species"=w203) -> (w205:T14)
        }
      }
    }
    "AFR Display" <- w136
    n75 = local read "Rig Temperatures"() -> (w116:T2)
    n76 = control-ref of="Rig Temperatures"() -> (w112:refnum<vi>)
    n77 = control-ref of="Rig Alarm Thresholds"() -> (w110:refnum<vi>)
    n78 = property class="Clust (strict)"(reference=w110) -> ("Controls[]"=w109:refnum<vi>[])  [unwired: 1 in, 2 out]
    n79 = property class="Clust (strict)"(reference=w112) -> ("Controls[]"=w111:refnum<vi>[])  [unwired: 1 in, 2 out]
    n80 = Cluster To Array(cluster=w116) -> (array=w113:dbl[])
    n81 = Cluster To Array(cluster="Rig Alarm Thresholds") -> (array=w115:dbl[])
    n82 = Array Size(array=w113) -> (size(s)=w114:i32)
    n83 = for {
      N: w114 -> [_]
      tunnel: w115 -> [w147] mode=indexing
      tunnel: w113 -> [w148] mode=indexing
      tunnel: w111 -> [w145] mode=indexing
      tunnel: w109 -> [w146] mode=indexing
      n84 = Greater?(x=w148, y=w147) -> (0:w144:bool)
      n85 = property on="Property Node" class="Ctl"(reference=w146, "Blinking"=w144) -> ()  [unwired: 1 in, 2 out]
      n86 = property on="Property Node" class="Ctl"(reference=w145, "Blinking"=w144) -> ()  [unwired: 1 in, 2 out]
    }
    n87 = Array To Cluster(array=w124) -> (cluster=→"Line Pressures":T3)
    n88 = Array To Cluster(array=w127) -> (cluster=→"Line Temperatures":T3)
    n89 = Get Date/Time In Seconds() -> (seconds since 1Jan1904=→"UI Timestamp":timestamp)
    n90 = Add Array Elements(numeric array=w120) -> (sum=w107:dbl)
    "Total Air Flow [g/s]" <- w107
    n91 = Add Array Elements(numeric array=w121) -> (sum=w125:dbl)
    "Total Fuel Flow [g/s]" <- w125
    n92 = Add Array Elements(numeric array=w122) -> (sum=w108:dbl)
    "Total Air Flow Required for \nStoichiometric Combustion" <- w108
    n93 = Add Array Elements(numeric array=w101) -> (sum=→"Thermal Power [kJ/s]":dbl)
    n94 = Divide(x=w108, y=w125) -> (x/y=→"Mixture AFR":dbl)
    n95 = Divide(x=w107, y=w108) -> (x/y=→"Equivalence Ratio":dbl)
  }
  n96 = while {
    shift-right: [w213] -> _
    shift-left: T7."Waiting to record" -> [w212]
    tunnel: w6 -> [w210]
    shift-right: [w208] -> _
    shift-left: _ -> [w209]
    shift-right: [w207] -> w5
    shift-left: _ -> [w206]
    stop <- w211 stop-if-true
    # "Output to File Loop"
    n97 = case shown="\"Recording\"" w212 {
      tunnel: [w218 w224 w246 T7."Finished Recording"] -> w213
      tunnel: [FALSE _ _ TRUE] -> w211
      tunnel: w210 -> [w214 _ w243 _]
      tunnel: w209 -> [w216 _ w240 w267]
      tunnel: [w216 w232 w241 w267] -> w208
      tunnel: [w215 w226 w236 w266] -> w207
      tunnel: w206 -> [w215 _ w239 w266]
      frame "Waiting to record", Default {
        n98 = call <extravilib>:"Read.vi"("channel"=w214) -> ()  [unwired: 6 in, 5 out]
        n99 = Select(t=T7."Creating Spreadsheet", s="Start Recording?", f=T7."Waiting to record") -> (s? t:f=w218:T7)
      }
      frame "Creating Spreadsheet" {
        n100 = call "Create Spreadsheet Headers for v3.2.vi"() -> ("Array"=w231:string[])  [unwired: 11 in]
        n101 = call-poly <vilib>:"Write Delimited Spreadsheet.vi"("file path (dialog if empty)"="file path (dialog if empty)", "1D data"=w231, "append to file? (new file:F)"=FALSE, "delimiter (\\t)"="," ("delimiter (\\t)")) -> ("new file path (Not A Path if cancelled)"=w232:path, "error out"=w227:errorcluster)  [unwired: 10 in]
        n102 = call <vilib>:"General Error Handler.vi"("error in (no error)"=w227) -> ("error?"=w225:bool, "error out"=w226:errorcluster)  [unwired: 10 in, 3 out]
        n103 = Select(t=T7."Waiting to record", s=w225, f=T7."Recording") -> (s? t:f=w224:T7)
      }
      frame "Recording" {
        n104 = local read "Actual Sample Rate"() -> (w233:dbl)
        n105 = for {
          N: w233 -> [_]
          tunnel: w243 -> [w264]
          tunnel: [w263] -> w242
          tunnel: [w248] -> w234 mode=indexing
          w253 = "," ("delimiter (Tab)")
          n106 = call <extravilib>:"Read.vi"("channel"=w264) -> ("done?"=w263:bool, "element"=w261:T10)  [unwired: 6 in, 3 out]
          n107 = Unbundle By Name(w261) -> ("Flowrate Data"=w262:T4, "DAQmx Data"=w259:dbl[], "Rig Temperatures"=w265:T11)
          n108 = Unbundle By Name(w261) -> ("Current Time"=w254:timestamp)
          "Export Timestamp" <- w254
          n109 = Cluster To Array(cluster=w265) -> (array=w260:dbl[])
          n110 = call "line flow cluster to 1d array.vi"("Flowrate Data"=w262) -> ("Array"=w258:dbl[])
          n111 = Build Array (concatenate)(w258, w259, w260) -> (w251:dbl[])
          n112 = Format Date/Time String(time format string (%c)="%d-%m-%y, %H:%M:%S%3u", seconds (now)=w254) -> (date/time string=w252:string)  [unwired: 1 in]
          n113 = Array To Spreadsheet String(delimiter (Tab)=w253, array=w251, 3:"%.3s" ("format string")) -> (spreadsheet string=w257:string)
          n114 = call <vilib>:"Trim Whitespace.vi"("string"=w257) -> ("trimmed string"=w249:string)  [unwired: 1 in]
          n115 = Concatenate Strings(w252, w253) -> (w250:string)
          n116 = Build Array(w250, w249) -> (w248:string[])
        }
        n117 = property on="Start Recording?" class="Bool"("DisabledEnum"=T9."Disabled and Grayed Out" ("Disabled")) -> ()  [unwired: 2 in, 2 out]
        n118 = property on="Stop Recording?" class="Bool"("DisabledEnum"=T9."Enabled" ("Disabled")) -> ()  [unwired: 2 in, 2 out]
        n119 = call-poly <vilib>:"Write Delimited Spreadsheet.vi"("file path (dialog if empty)"=w240, "format (%s)"="%s", "2D data"=w234, "append to file? (new file:F)"=TRUE, "error in (no error)"=w239) -> ("new file path (Not A Path if cancelled)"=w241:path, "error out"=w236:errorcluster)  [unwired: 9 in]
        n120 = Select(t=T7."Finished Recording", s=w242, f=T7."Recording") -> (s? t:f=w246:T7)
      }
      frame "Finished Recording" {
      }
    }
    "Export Loop Status" <- w213
  }
  n121 = call <vilib>:"General Error Handler.vi"("error in (no error)"=w5) -> ()  [unwired: 10 in, 5 out]
